vi "ExampleInitHelper.vi"(7 "Device Config Name":string="testconfig_qmixsdk") -> (2 "Plugin Search Path":string, 3 "Device Configuration Path":string)   [LabVIEW 2021]
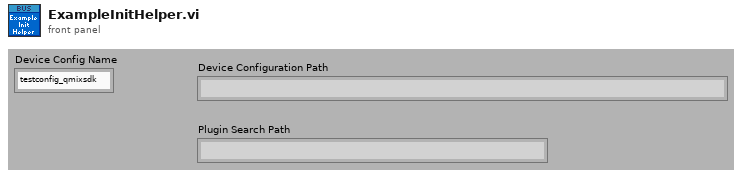
[diagram p1: front panel]
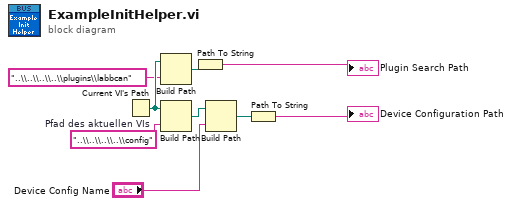
[diagram p0: block diagram]
diagram:
  n1 = Current VI's Path "Pfad des aktuellen VIs"() -> (path=w8:path)
  n2 = Build Path(base path=w8, name or relative path="..\\..\\..\\..\\plugins\\labbcan" ("Name oder relativer Pfad")) -> (appended path=w6:path)
  n3 = Build Path(base path=w8, name or relative path="..\\..\\..\\..\\config" ("Name oder relativer Pfad")) -> (appended path=w3:path)
  n4 = Path To String(path=w6) -> (string=→"Plugin Search Path":string)
  n5 = Build Path(base path=w3, name or relative path="Device Config Name") -> (appended path=w2:path)
  n6 = Path To String(path=w2) -> (string=→"Device Configuration Path":string)
